vi "Pack Notification Message Adapter.vi"(10 "Message":refnum<class "Message.lvclass">) -> (3 "NotificationMessageAdapter":refnum<class "NotificationMessageAdapter.lvclass">)   [LabVIEW 2017, in "ActorMessageTransport.lvlib" / "NotificationMessageAdapter.lvclass"]
uses:
  NotificationMessageAdapter.lvclass
  <vilib>/ActorFramework/Message/Message.lvclass
  NotificationMessageAdapter.lvclass/NotificationMessageAdapter.ctl
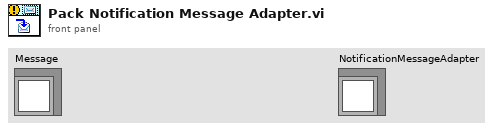
[diagram p1: front panel]
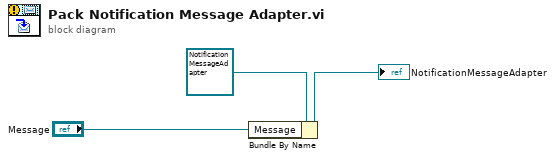
[diagram p0: block diagram]
diagram:
  n1 = Bundle By Name(cluster=refnum<class "NotificationMessageAdapter.lvclass"> refnum ("NotificationMessageAdapter"), "Message"="Message") -> (→"NotificationMessageAdapter":refnum<class "NotificationMessageAdapter.lvclass">)
